vi "Event Nested.vi"(8 "Alias":string, 10 "Event":refnum<class "Event.lvclass">, 11 "jettl Queue Actor in":refnum<class "jettl Queue Actor.lvclass">) -> (3 "jettl Queue Actor out":refnum<class "jettl Queue Actor.lvclass">)   [LabVIEW 2021, in "jettl.lvlib" / "jettl Queue Actor.lvlib" / "jettl Queue Actor.lvclass"]
uses:
  jettl Queue Actor.lvclass
  jettl Queue Actor.lvclass/jettl Queue Actor.ctl
  Actor/Event/Event.lvclass
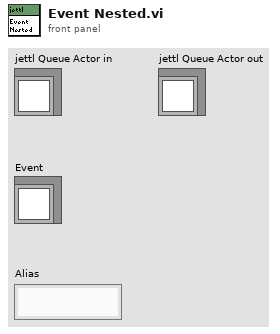
[diagram p1: front panel]
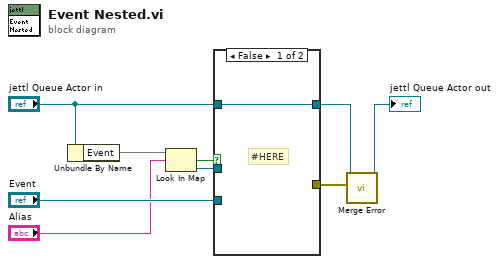
[diagram p0: block diagram]
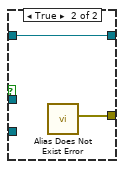
[diagram p2: hidden frame]
diagram:
  n1 = Unbundle By Name("jettl Queue Actor in") -> ("Event"=w9:map{string, refnum<data-value>})
  n2 = Look In Map(map=w9, key="Alias") -> (key not found?=w8:bool, value=w2:refnum<data-value>)  [unwired: 1 in]
  n3 = case shown="False" w8 {
    tunnel: [_ w12] -> w7
    tunnel: "Event" -> [_ _]
    tunnel: w2 -> [_ _]
    tunnel: [w10 w11] -> w4
    tunnel: "jettl Queue Actor in" -> [w10 w11]
    frame False {
      # "#HERE"
    }
    frame True {
      n4 = call "Alias Does Not Exist Error.vi"() -> ("Error"=w12:errorcluster)  [unwired: 11 in]
    }
  }
  n5 = call-dynamic "Merge Error.vi"("Error"=w7, "jettl Queue Actor in"=w4) -> ("jettl Queue Actor out"=→"jettl Queue Actor out":refnum<class "jettl Queue Actor.lvclass">)  [unwired: 9 in]
